vi "- VI Tree - Variant XML.vi"   [LabVIEW 2011]
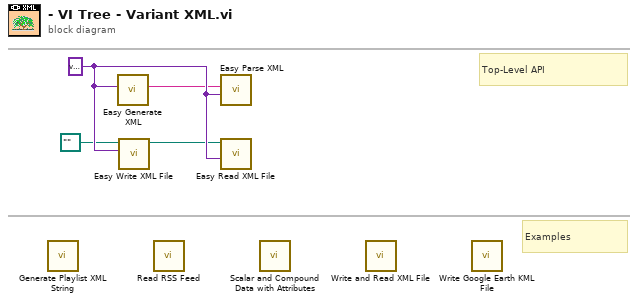
[diagram p0: block diagram]
diagram:
  w4 = variant ("LabVIEW Data")
  # "Examples"
  # "Top-Level API"
  n1 = call "Generate Playlist XML String.vi"() -> ()  [unwired: 1 in]
  n2 = call "Easy Generate XML.vi"("LabVIEW Data"=w4) -> ("XML String"=w3:string)  [unwired: 9 in, 1 out]
  n3 = call "Easy Write XML File.vi"("LabVIEW Data"=w4, "XML File Path"=path "") -> ("XML File Path (duplicate)"=w1:path)  [unwired: 8 in, 1 out]
  n4 = call "Read RSS Feed.vi"() -> ()  [unwired: 1 in]
  n5 = call "Easy Parse XML.vi"("LabVIEW Data (Type)"=w4, "XML String"=w3) -> ()  [unwired: 8 in, 2 out]
  n6 = call "Easy Read XML File.vi"("LabVIEW Data (Type)"=w4, "XML File Path"=w1) -> ()  [unwired: 7 in, 3 out]
  n7 = call "Scalar and Compound Data with Attributes.vi"() -> ()  [unwired: 1 in]
  n8 = call "Write and Read XML File.vi"() -> ()  [unwired: 1 in]
  n9 = call "Write Google Earth KML File.vi"() -> ()  [unwired: 1 in]
